vi "DARPA_DoubleJ_20220715_Arduino_ver.vi"() -> ()   [LabVIEW 2021]
uses:
  <vilib>/rvi/interface/nirviReadWriteControl/nirviReadWriteControl.xnode
  <vilib>/rvi/interface/nirviOpenFPGA/nirviOpenFPGA.xnode
  <vilib>/rvi/interface/nirviCloseFPGA/nirviCloseFPGA.xnode
  <vilib>/Instr/_visa.llb/VISA Configure Serial Port (Instr).vi
  NiFpgaLv.dll
  <vilib>/Utility/error.llb/Error Cluster From Error Code.vi
  <vilib>/rvi/interface/Simulation/niFpgaSimulationCallBeginRW.vi
  <vilib>/rvi/errors/niLvFpgaAdjustHostInterfaceError.vi
  <vilib>/FPGAPlugInAG/Dynamic/niLvFpga_Close_Dynamic.vi
  FPGA Bitfiles/darpatransitionj_FPGATarget_DARPAFPGADoubleJ_E+A750Kw4Ow.lvbitx
  DARPA_FPGA_DoubleJ_20220715.vi
  <vilib>/FPGAPlugInAG/PCIe-7857/niLvFpga_Open_PCIe-7857.vi
  <vilib>/rvi/interface/common/dynamic/niFpgaDynamicAddResources.vi
panel:
  in  "ratiocontrol":dbl
  in  "Arduino COM port":refnum<visa-resource-name>="COM7"
  in  "Shut down program 2":bool=TRUE
  in  "Initializer":bool
  out "read":string
  in  "PMT2 senstivity":bool
  in  "PMT1 senstivity":bool
  in  "Func amp":bool
  in  "Func Freq":bool
  in  "Func On time":bool
  in  "Func Delay":bool
  in  "PMT1 senstivity input":dbl caption="0.5-0.75 V"
  in  "PMT2 senstivity input":dbl caption="0.5-0.75 V"
  in  "Func amp input":dbl caption="0 - 5 V"
  in  "Func freq input":dbl caption="100 - 10k Hz"
  in  "Func on Time input":dbl caption="0.01 - 1 s"
  in  "Func delay input":dbl caption="0.01 - 1 s"
  out "PMT2 sum":u64(graph)
  out "PMT1 sum":u64(graph)
  out "Unfiltered Signal 1":i16(graph)
  out "Filtered Signal 2":i16(graph)
  out "Unfiltered Signal 2":i16(graph)
  in  "Threshold1":dbl=2.0
  in  "Threshold2":dbl=1.0
  out "LabView Timer (sec)":dbl
  out "sample diff":u64
  out "t1 (sample)":u64
  out "t0 (sample)":u64
  out "PMT1 sum":u64
  out "PMT2 sum":u64
  out "Droplet lock on":bool
  out "Filtered Signal1":dbl
  out "Filtered Signal2":dbl
  out "Droplet counter":u64
  out "Unfiltered Signal1":dbl
  out "Unfiltered Signal2":dbl
  in  "Droplet width [ms]":dbl=5.0
  in  "determine ratio (xx.xx)":dbl=1.0
  out "FPGA loop counter":u64
  out "Sorted droplet counter":u64
  out "Sort":bool
  in  "FPGA initializer":bool=TRUE
  out "FPGA timer (sec)":dbl
  out "FPGA freq":dbl
  out "LabView freq":dbl
  out "Filtered Signal 1":i16(graph)
  out "PMT1/PMT2":dbl
  out "PMT1/PMT2 (graph)":dbl(graph)
  in  "Shut down program":bool=TRUE
  in  "Set rate1":dbl=1000.0 format="%#_4g"
  in  "Units1":string(combo)="uh"
  in  "Target Vol1":dbl=1000.0 caption="Target Vol (ul)"
  in  "Direction1":string(combo)="inf"
  in  "Send1":bool
  out "Max rate1":dbl format="%#_4g"
  out "Min rate1":dbl caption="Min rate" format="%#_4g"
  in  "Pump1\nStart/Stop":bool
  out "Dispensed1":string
  in  "Reset1":bool
  out "Remains1":string
  in  "Syringe Selection1":string(combo)="BDP1MM"
  in  "dia1 (mm)":dbl=0.1 caption="Set Diameter (mm)" min=0.1 max=50.0
  out "Diameter1 (mm)":dbl
  in  "Set rate2":dbl format="%#_4g"
  in  "Units2":string(combo)="mm"
  in  "Target Vol2":dbl caption="Target Vol (ul)"
  in  "Direction2":string(combo)="inf"
  out "Max rate2":dbl format="%#_4g"
  out "Min rate2":dbl caption="Min rate" format="%#_4g"
  in  "Syringe Selection2":string(combo)="CUS"
  in  "dia2 (mm)":dbl=0.1 caption="Set Diameter (mm)" min=0.1 max=50.0
  out "Diameter2 (mm)":dbl
  in  "Set rate3":dbl format="%#_4g"
  in  "Units3":string(combo)="mm"
  in  "Target Vol3":dbl caption="Target Vol (ul)"
  in  "Direction3":string(combo)="inf"
  out "Max rate3":dbl format="%#_4g"
  out "Min rate3":dbl caption="Min rate" format="%#_4g"
  in  "Syringe Selection3":string(combo)="CUS"
  in  "dia3 (mm)":dbl=0.1 caption="Set Diameter (mm)" min=0.1 max=50.0
  out "Diameter3 (mm)":dbl
  in  "Set rate4":dbl format="%#_4g"
  in  "Units4":string(combo)="mm"
  in  "Target Vol4":dbl caption="Target Vol (ul)"
  in  "Direction4":string(combo)="inf"
  out "Max rate4":dbl format="%#_4g"
  out "Min rate4":dbl caption="Min rate" format="%#_4g"
  in  "Syringe Selection4":string(combo)="CUS"
  in  "dia4 (mm)":dbl=0.1 caption="Set Diameter (mm)" min=0.1 max=50.0
  out "Diameter4 (mm)":dbl
  in  "Pump2\nStart/Stop":bool
  in  "Pump3\nStart/Stop":bool
  in  "Pump4\nStart/Stop":bool
  out "Dispensed2":string
  out "Dispensed3":string
  out "Dispensed4":string
  out "Remains2":string
  out "Remains3":string
  out "Remains4":string
  in  "Reset2":bool
  in  "Reset3":bool
  in  "Reset4":bool
  in  "Syringe COM port":refnum<visa-resource-name>="COM3"
  out "Baud Rate":string
  in  "Output file path":string="D:\\PhD\\00TAMU\\1.research\\nanoBioSystem\\1.projects\\1.DARPA_iSENTRY\\2.src\\LabView\\transition\\FPGA7857\\output file"
  in  "file name":string="FullyAlive1"
  out "Confirm path":string
  out "Data File Ptr":refnum<file>
  # "For inner peace of developers"
  # "Communication Setting"
  # "Sorting Status"
  # "Hammamatsu display"
  # "[Pump1] Syringe Setting"
  # "[Pump2] Syringe Setting"
  # "PMT display"
  # "[Pump3] Syringe Setting"
  # "[Pump4] Syringe Setting"
  # "File saving option"
  # "Cockpit"
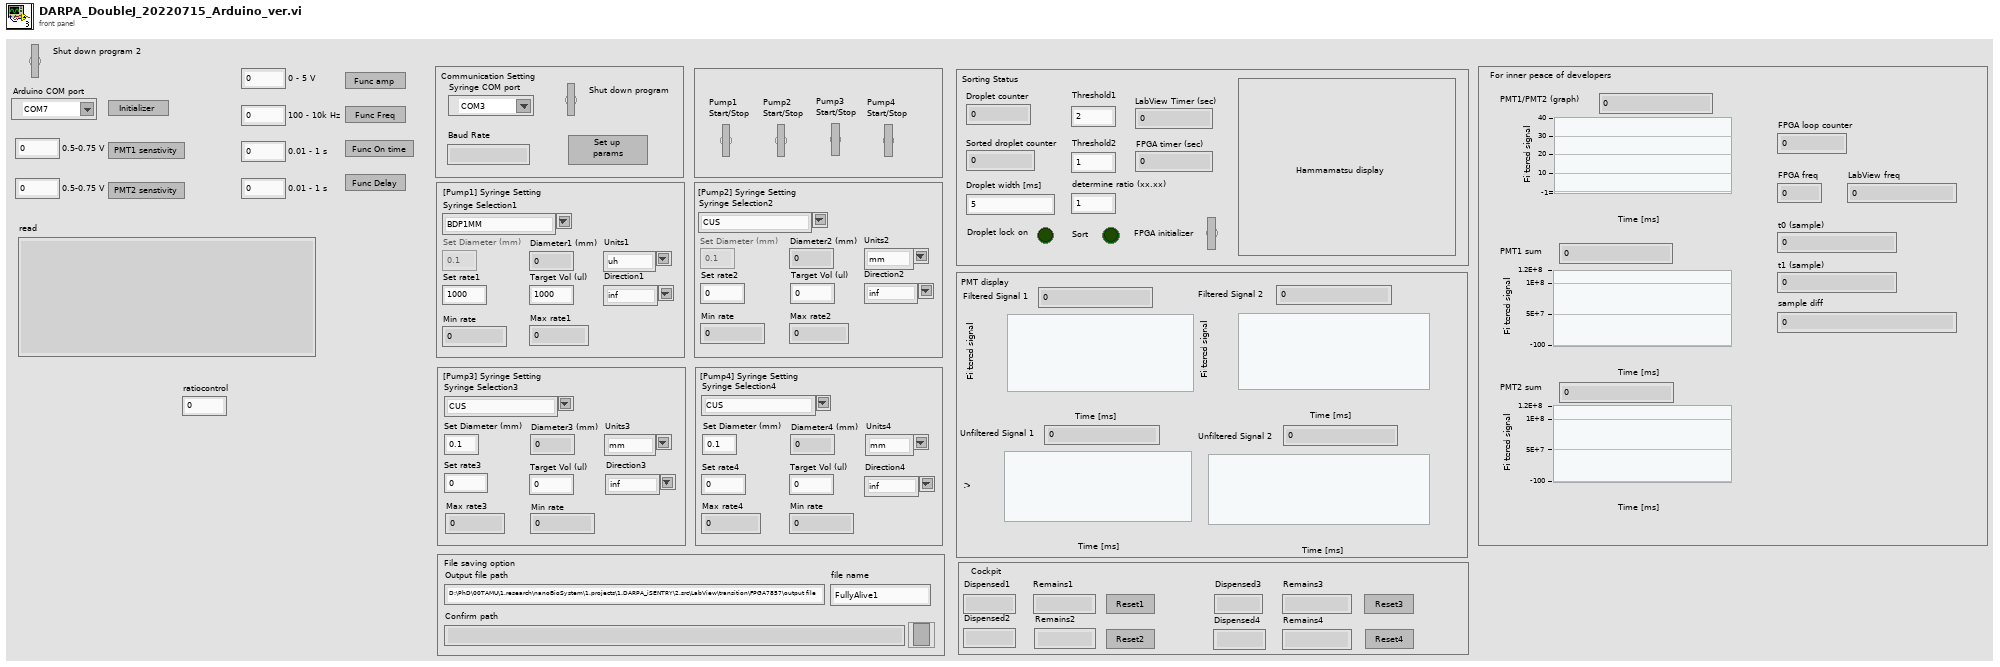
[diagram p1: front panel]
types:
  T1 = enum16{"open", "replace", "create", "open or create", "replace or create", "replace or create with confirmation"}
  T2 = enum8{"Enabled", "Disabled", "Disabled and Grayed Out"}
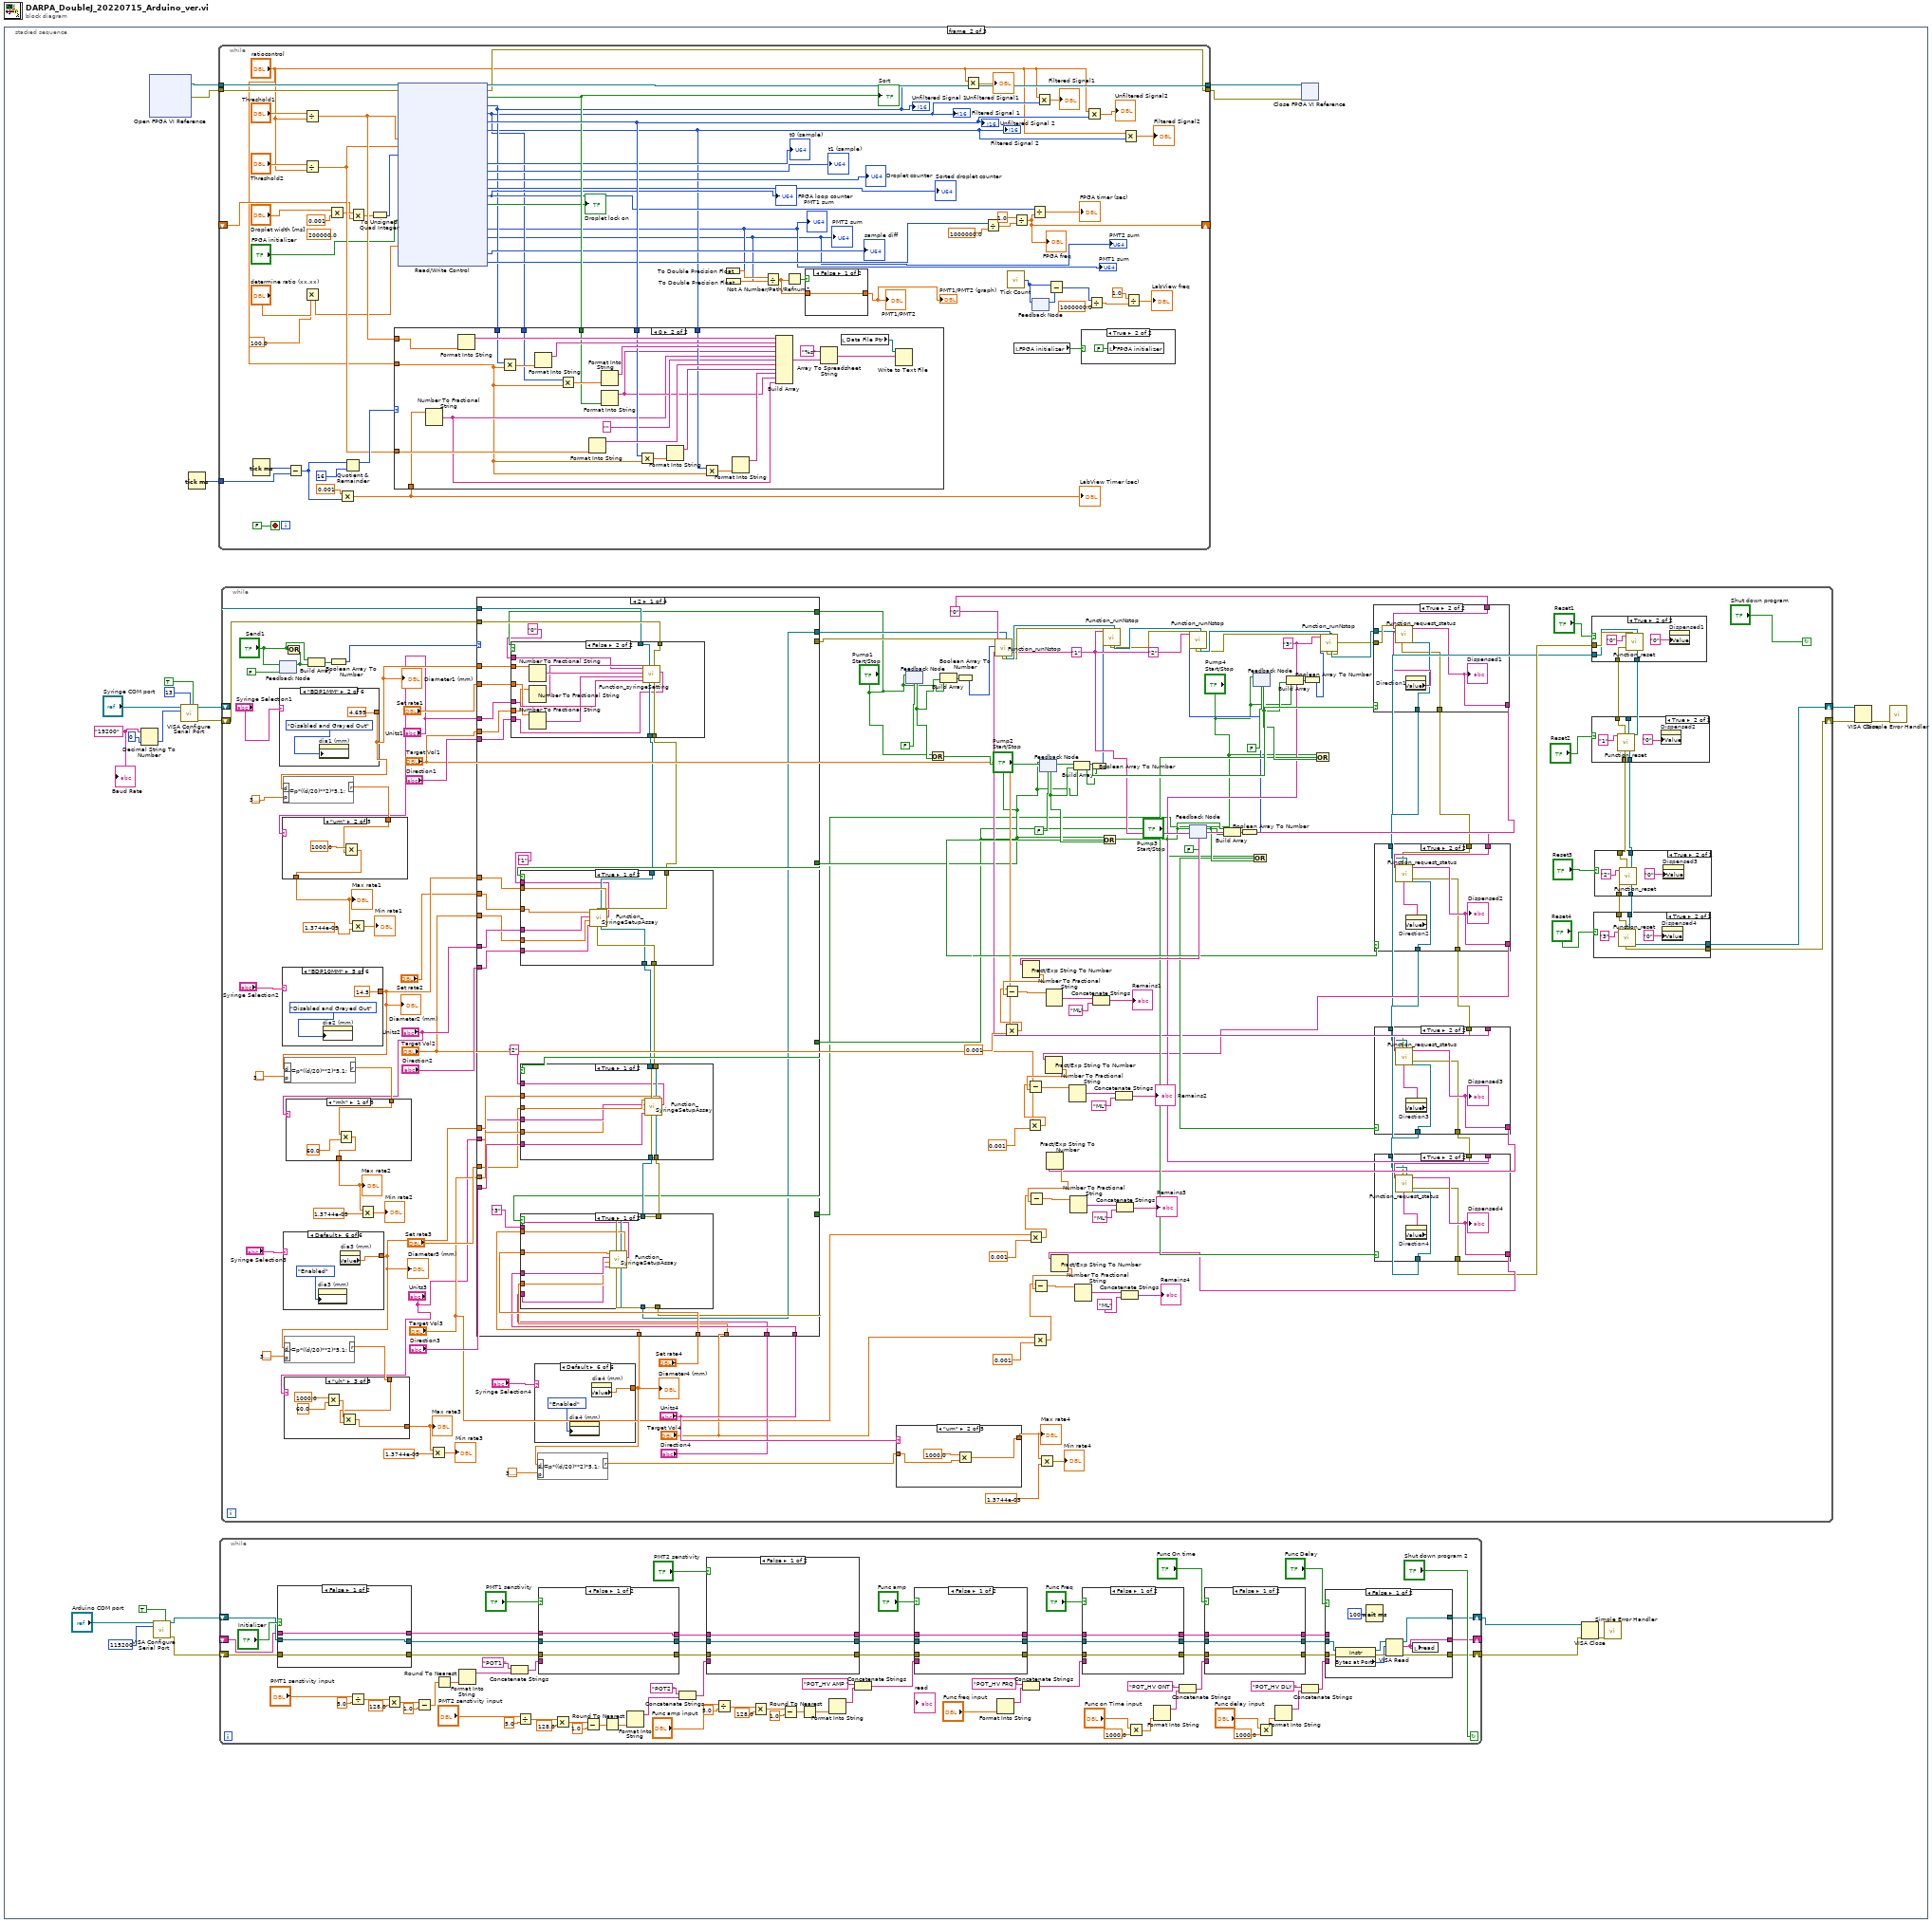
[diagram p0: block diagram]
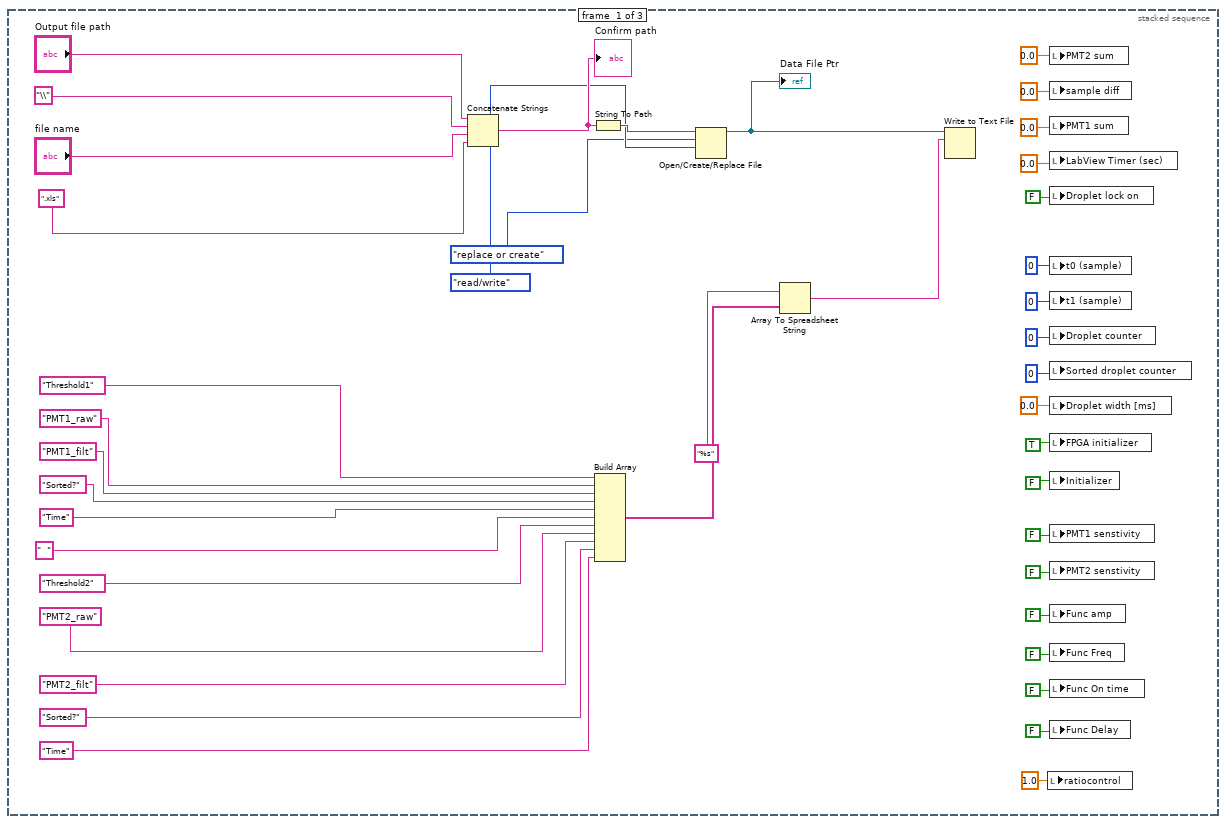
[diagram p2: hidden frame]
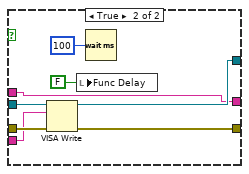
[diagram p3: hidden frame]
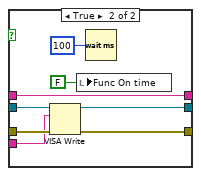
[diagram p4: hidden frame]
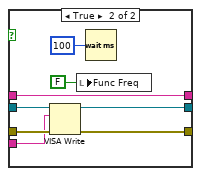
[diagram p5: hidden frame]
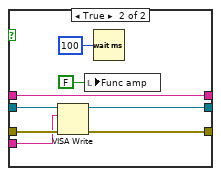
[diagram p6: hidden frame]
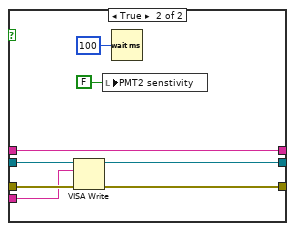
[diagram p7: hidden frame]
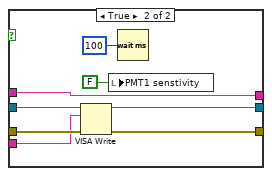
[diagram p8: hidden frame]
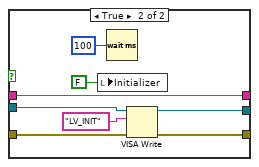
[diagram p9: hidden frame]
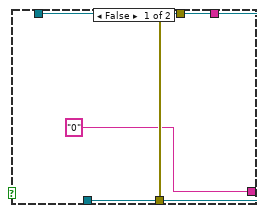
[diagram p14: hidden frame]
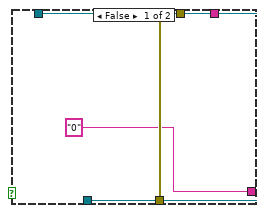
[diagram p15: hidden frame]
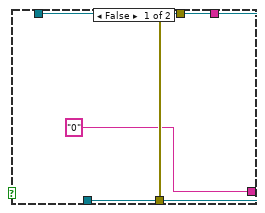
[diagram p16: hidden frame]
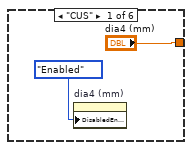
[diagram p17: hidden frame]
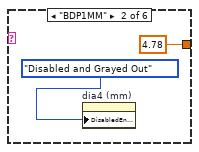
[diagram p18: hidden frame]
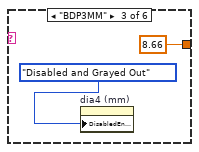
[diagram p19: hidden frame]
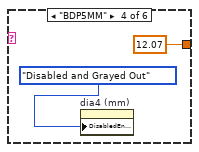
[diagram p20: hidden frame]
diagram:
  n1 = stacked-sequence {
    frame #0 {
      n2 = Concatenate Strings("Output file path", "\\" ("string"), "file name", ".xls" ("string")) -> (w41:string)
      "Confirm path" <- w41
      n3 = String To Path(string=w41) -> (path=w42:path)
      n4 = Build Array("Threshold1", "PMT1_raw", "PMT1_filt", "Sorted?", "Time", "  ", "Threshold2", "PMT2_raw", "PMT2_filt", "Sorted?", "Time") -> (w34:string[])
      n5 = Open/Create/Replace File(file path (use dialog)=w42, operation (0:open)=T1."replace or create", access (0:read/write)=enum16{"read/write", "read-only", "write-only"}."read/write") -> (refnum out=w20:refnum<file>)  [unwired: 3 in, 2 out]
      "Data File Ptr" <- w20
      n6 = Array To Spreadsheet String(array=w34, 3:"%s") -> (spreadsheet string=w22:string)  [unwired: 1 in]
      n7 = Write to Text File(file (use dialog)=w20, text=w22) -> ()  [unwired: 2 in, 3 out]
      n8 = local write "ratiocontrol"(1.0 ("ratiocontrol")) -> ()
      n9 = local write "PMT2 sum"(0.0 ("now")) -> ()
      n10 = local write "sample diff"(0.0 ("sample diff")) -> ()
      n11 = local write "PMT1 sum"(0.0 ("PMT1 sum")) -> ()
      n12 = local write "LabView Timer (sec)"(0.0 ("PMT2 sum")) -> ()
      n13 = local write "Droplet lock on"(FALSE ("Droplet lock on")) -> ()
      n14 = local write "t0 (sample)"(u64 0 ("t0 (sample)")) -> ()
      n15 = local write "t1 (sample)"(u64 0 ("t1 (sample)")) -> ()
      n16 = local write "Droplet counter"(u64 0 ("Droplet counter")) -> ()
      n17 = local write "Sorted droplet counter"(u64 0 ("Sorted droplet counter")) -> ()
      n18 = local write "Droplet width [ms]"(0.0 ("Time compensation [ms]")) -> ()
      n19 = local write "FPGA initializer"(TRUE ("FPGA initializer")) -> ()
      n20 = local write "Initializer"(FALSE ("FPGA initializer")) -> ()
      n21 = local write "PMT1 senstivity"(FALSE ("FPGA initializer")) -> ()
      n22 = local write "PMT2 senstivity"(FALSE ("FPGA initializer")) -> ()
      n23 = local write "Func amp"(FALSE ("FPGA initializer")) -> ()
      n24 = local write "Func Freq"(FALSE ("FPGA initializer")) -> ()
      n25 = local write "Func On time"(FALSE ("FPGA initializer")) -> ()
      n26 = local write "Func Delay"(FALSE ("FPGA initializer")) -> ()
    }
    frame #1 {
      w56 = "19200" ("Baud Rate")
      n27 = Decimal String To Number(string=w56, default (0L)=u32 0 ("default (0 I32)")) -> (number=w59:u32)  [unwired: 1 in, 1 out]
      n28 = xnode "Open FPGA VI Reference"() -> ("FPGA VI Reference Out"=w66:refnum<k20>, "error out"=w65:errorcluster)  [unwired: 2 in]
      n29 = call-poly "VISA Configure Serial Port"("VISA resource name"="Arduino COM port", "Enable Termination\nChar (T)"=TRUE ("Enable Termination\nChar (T)"), "baud rate (9600)"=u32 115200) -> ("VISA resource name out"=w46:refnum<visa-resource-name>, "error out"=w45:errorcluster)  [unwired: 11 in]
      n30 = call-poly "VISA Configure Serial Port"("VISA resource name"="Syringe COM port", "termination char\n(0xA = '\\n' = LF)"=u8 13 ("termination char\n(0xA = '\\n' = LF)"), "Enable Termination\nChar (T)"=TRUE ("Enable Termination\nChar (T)"), "baud rate (9600)"=w59) -> ("VISA resource name out"=w55:refnum<visa-resource-name>, "error out"=w54:errorcluster)  [unwired: 10 in]
      n31 = Tick Count (ms)() -> (millisecond timer value=w62:u32)
      n32 = while {
        tunnel: w66 -> [w744]
        tunnel: [w743] -> w64
        tunnel: w65 -> [w742]
        tunnel: [w741] -> w63
        tunnel: w62 -> [w739]
        shift-right: [w683] -> _
        shift-left: _ -> [w682]
        stop <- FALSE stop-if-true
        (unwired) 200000.0 ("y")
        n33 = Tick Count (ms)() -> (millisecond timer value=w738:u32)
        n34 = Subtract(x=w738, y=w739) -> (x-y=w733:u32)
        n35 = Divide(x="Threshold1", y="ratiocontrol") -> (x/y=w726:dbl)
        n36 = Divide(x="Threshold2", y="ratiocontrol") -> (x/y=w725:dbl)
        n37 = Multiply(x="determine ratio (xx.xx)", y=100.0) -> (x*y=w706:dbl)
        n38 = Multiply(x="Droplet width [ms]", y=0.001) -> (x*y=w708:dbl)
        n39 = Multiply(x=0.001, y=w733) -> (x*y=w700:dbl)
        "LabView Timer (sec)" <- w700
        n40 = Quotient & Remainder(x=w733, y=u32 16) -> (x-y*floor(x/y)=w735:u32)  [unwired: 1 out]
        n41 = Multiply(x=w708, y=w682) -> (x*y=w707:dbl)
        n42 = To Unsigned Quad Integer(1:w707) -> (0:w721:u64)
        n43 = xnode "Read/Write Control"("FPGA VI Reference In"=w744, "error in"=w742, "Threshold1"=w726, "Threshold2"=w725, "Time compensation [clock]"=w721, "FPGA initializer"="FPGA initializer", "determine ratio"=w706) -> ("FPGA VI Reference Out"=w743:refnum<k20>, "error out"=w741:errorcluster, "Sort"=w724:bool, "Unfiltered  Signal1"=w703:i16, "Filtered Signal1"=w691:i16, "Unfiltered  Signal2"=w727:i16, "Filtered Signal2"=w702:i16, "t0 (sample)"=→"t0 (sample)":u64, "t1 (sample)"=→"t1 (sample)":u64, "Droplet counter"=→"Droplet counter":u64, "Sorted droplet counter"=→"Sorted droplet counter":u64, "loop counter"=w712:u64, "Droplet lock on"=→"Droplet lock on":bool, "PMT1 sum"=w685:u64, "PMT2 sum"=w684:u64, "sample diff"=→"sample diff":u64, "Loop length (uSec)"=w711:u32)  [unwired: 1 out]
        "Unfiltered Signal 1" <- w703
        "Filtered Signal 2" <- w702
        "Unfiltered Signal 2" <- w727
        "PMT1 sum" <- w685
        "PMT2 sum" <- w684
        "FPGA loop counter" <- w712
        "Sort" <- w724
        "Filtered Signal 1" <- w691
        "PMT1 sum" <- w685
        "PMT2 sum" <- w684
        n44 = case shown="0" w735 {
          tunnel: w727 -> [_ w760]
          tunnel: w702 -> [_ w759]
          tunnel: w691 -> [_ w758]
          tunnel: w703 -> [_ w757]
          tunnel: w725 -> [_ w755]
          tunnel: w726 -> [_ w754]
          tunnel: w724 -> [_ w752]
          tunnel: w700 -> [_ w750]
          tunnel: "ratiocontrol" -> [_ w748]
          frame Default {
          }
          frame 0 {
            n45 = Number To Fractional String(number=w750) -> (F-format string=w749:string)  [unwired: 3 in]
            n46 = Format Into String(w754) -> (resulting string=w762:string)  [unwired: 3 in, 1 out]
            n47 = Multiply(x=w757, y=w748) -> (x*y=w770:dbl)
            n48 = Format Into String(w770) -> (resulting string=w761:string)  [unwired: 3 in, 1 out]
            n49 = Multiply(x=w758, y=w748) -> (x*y=w771:dbl)
            n50 = Format Into String(w755) -> (resulting string=w764:string)  [unwired: 3 in, 1 out]
            n51 = Format Into String(w771) -> (resulting string=w763:string)  [unwired: 3 in, 1 out]
            n52 = Format Into String(w752) -> (resulting string=w751:string)  [unwired: 3 in, 1 out]
            n53 = Multiply(x=w760, y=w748) -> (x*y=w772:dbl)
            n54 = Format Into String(w772) -> (resulting string=w765:string)  [unwired: 3 in, 1 out]
            n55 = Multiply(x=w759, y=w748) -> (x*y=w773:dbl)
            n56 = Format Into String(w773) -> (resulting string=w766:string)  [unwired: 3 in, 1 out]
            n57 = Build Array(w762, w761, w763, w751, w749, "" ("element"), w764, w765, w766, w751, w749) -> (w768:string[])
            n58 = Array To Spreadsheet String(array=w768, 3:"%s" ("format string")) -> (spreadsheet string=w767:string)  [unwired: 1 in]
            n59 = local read "Data File Ptr"() -> (w769:refnum<file>)
            n60 = Write to Text File(file (use dialog)=w769, text=w767) -> ()  [unwired: 2 in, 3 out]
          }
        }
        n61 = To Double Precision Float(number=w685) -> (double precision float=w690:dbl)
        n62 = To Double Precision Float(number=w684) -> (double precision float=w689:dbl)
        n63 = Divide(x=w690, y=w689) -> (x/y=w686:dbl)
        n64 = Not A Number/Path/Refnum?(number/path/refnum=w686) -> (NaN/Path/Refnum?=w688:bool)
        n65 = case shown="False" w688 {
          tunnel: [w745 0.0] -> w687
          tunnel: w686 -> [w745 _]
          frame False {
          }
          frame True {
          }
        }
        "PMT1/PMT2" <- w687
        "PMT1/PMT2 (graph)" <- w687
        n66 = Multiply(x="ratiocontrol", y=w703) -> (x*y=→"Unfiltered Signal1":dbl)
        n67 = Divide(x=w711, y=1000000.0 ("x")) -> (x/y=w709:dbl)
        n68 = call "Tick Count"() -> ("Tick Count(uSec)"=w693:u32)
        n69 = Divide(x=1.0, y=w709) -> (x/y=w683:dbl)
        "FPGA freq" <- w683
        n70 = local read "FPGA initializer"() -> (w713:bool)
        n71 = Divide(x=w712, y=w683) -> (x/y=→"FPGA timer (sec)":dbl)
        n72 = feedback #1() -> (w692:u32)  [unwired: 1 in]
        n73 = feedback-in #1(w693) -> ()
        n74 = Multiply(x="ratiocontrol", y=w691) -> (x*y=→"Filtered Signal1":dbl)
        n75 = Subtract(x=w693, y=w692) -> (x-y=w694:u32)
        n76 = case shown="True" w713 {
          frame False {
          }
          frame True {
            n77 = local write "FPGA initializer"(FALSE ("FPGA initializer")) -> ()
          }
        }
        n78 = Multiply(x="ratiocontrol", y=w727) -> (x*y=→"Unfiltered Signal2":dbl)
        n79 = Divide(x=w694, y=1000000.0 ("x")) -> (x/y=w697:dbl)
        n80 = Multiply(x="ratiocontrol", y=w702) -> (x*y=→"Filtered Signal2":dbl)
        n81 = Divide(x=1.0, y=w697) -> (x/y=→"LabView freq":dbl)
      }
      n82 = while {
        shift-right: [w126] -> w43
        shift-left: w46 -> [w146]
        shift-right: [w125] -> w47
        shift-left: w45 -> [w145]
        shift-right: [w127] -> _
        shift-left: _ -> [w143]
        stop <- "Shut down program 2" continue-if-true
        n83 = case shown="False" "Initializer" {
          tunnel: w146 -> [w220 w230]
          tunnel: w145 -> [w221 w229]
          tunnel: [w220 w226] -> w142
          tunnel: [w221 w225] -> w141
          tunnel: w143 -> [w222 w224]
          tunnel: [w222 w224] -> w140
          frame False {
          }
          frame True {
            n84 = local write "Initializer"(FALSE ("send")) -> ()
            n85 = Wait (ms)(milliseconds to wait=u32 100) -> ()  [unwired: 1 out]
            n86 = VISA Write(VISA resource name=w230, write buffer="LV_INIT", error in (no error)=w229) -> (VISA resource name out=w226:refnum<visa-resource-name>, error out=w225:errorcluster)  [unwired: 1 out]
          }
        }
        n87 = Divide(x="PMT1 senstivity input", y=5.0) -> (x/y=w109:dbl)
        n88 = Multiply(x=w109, y=128.0) -> (x*y=w111:dbl)
        n89 = Subtract(x=w111, y=1.0) -> (x-y=w106:dbl)
        n90 = Round To Nearest(number=w106) -> (nearest integer value=w115:dbl)
        n91 = Format Into String(w115) -> (resulting string=w114:string)  [unwired: 3 in, 1 out]
        n92 = Concatenate Strings("POT1 " ("string"), w114) -> (w112:string)
        n93 = Divide(x="PMT2 senstivity input", y=5.0) -> (x/y=w101:dbl)
        n94 = case shown="False" "PMT1 senstivity" {
          tunnel: w142 -> [w210 w219]
          tunnel: w141 -> [w209 w218]
          tunnel: [w210 w215] -> w139
          tunnel: [w209 w214] -> w138
          tunnel: w140 -> [w211 w213]
          tunnel: [w211 w213] -> w137
          tunnel: w112 -> [_ w212]
          frame False {
          }
          frame True {
            n95 = VISA Write(VISA resource name=w219, write buffer=w212, error in (no error)=w218) -> (VISA resource name out=w215:refnum<visa-resource-name>, error out=w214:errorcluster)  [unwired: 1 out]
            n96 = local write "PMT1 senstivity"(FALSE ("send")) -> ()
            n97 = Wait (ms)(milliseconds to wait=u32 100) -> ()  [unwired: 1 out]
          }
        }
        n98 = Multiply(x=w101, y=128.0) -> (x*y=w99:dbl)
        n99 = Subtract(x=w99, y=1.0) -> (x-y=w103:dbl)
        n100 = Round To Nearest(number=w103) -> (nearest integer value=w96:dbl)
        n101 = Format Into String(w96) -> (resulting string=w97:string)  [unwired: 3 in, 1 out]
        n102 = Concatenate Strings("POT2 " ("string"), w97) -> (w94:string)
        n103 = case shown="False" "PMT2 senstivity" {
          tunnel: w139 -> [w198 w208]
          tunnel: w138 -> [w199 w207]
          tunnel: [w198 w204] -> w123
          tunnel: [w199 w203] -> w122
          tunnel: w137 -> [w200 w202]
          tunnel: [w200 w202] -> w124
          tunnel: w94 -> [_ w201]
          frame False {
          }
          frame True {
            n104 = VISA Write(VISA resource name=w208, write buffer=w201, error in (no error)=w207) -> (VISA resource name out=w204:refnum<visa-resource-name>, error out=w203:errorcluster)  [unwired: 1 out]
            n105 = local write "PMT2 senstivity"(FALSE ("send")) -> ()
            n106 = Wait (ms)(milliseconds to wait=u32 100) -> ()  [unwired: 1 out]
          }
        }
        n107 = Divide(x="Func amp input", y=5.0) -> (x/y=w88:dbl)
        n108 = Multiply(x=w88, y=128.0) -> (x*y=w90:dbl)
        n109 = Subtract(x=w90, y=1.0) -> (x-y=w86:dbl)
        n110 = Round To Nearest(number=w86) -> (nearest integer value=w92:dbl)
        n111 = Format Into String(w92) -> (resulting string=w91:string)  [unwired: 3 in, 1 out]
        n112 = Concatenate Strings("POT_HV AMP " ("string"), w91) -> (w84:string)
        n113 = case shown="False" "Func amp" {
          tunnel: w123 -> [w189 w197]
          tunnel: w122 -> [w187 w196]
          tunnel: [w189 w193] -> w136
          tunnel: [w187 w192] -> w135
          tunnel: w124 -> [w188 w191]
          tunnel: [w188 w191] -> w134
          tunnel: w84 -> [_ w190]
          frame False {
          }
          frame True {
            n114 = VISA Write(VISA resource name=w197, write buffer=w190, error in (no error)=w196) -> (VISA resource name out=w193:refnum<visa-resource-name>, error out=w192:errorcluster)  [unwired: 1 out]
            n115 = local write "Func amp"(FALSE ("send")) -> ()
            n116 = Wait (ms)(milliseconds to wait=u32 100) -> ()  [unwired: 1 out]
          }
        }
        n117 = Format Into String("Func freq input") -> (resulting string=w83:string)  [unwired: 3 in, 1 out]
        n118 = Concatenate Strings("POT_HV FRQ " ("string"), w83) -> (w80:string)
        n119 = case shown="False" "Func Freq" {
          tunnel: w136 -> [w177 w186]
          tunnel: w135 -> [w176 w185]
          tunnel: [w177 w182] -> w128
          tunnel: [w176 w181] -> w129
          tunnel: w134 -> [w178 w180]
          tunnel: [w178 w180] -> w133
          tunnel: w80 -> [_ w179]
          frame False {
          }
          frame True {
            n120 = VISA Write(VISA resource name=w186, write buffer=w179, error in (no error)=w185) -> (VISA resource name out=w182:refnum<visa-resource-name>, error out=w181:errorcluster)  [unwired: 1 out]
            n121 = local write "Func Freq"(FALSE ("send")) -> ()
            n122 = Wait (ms)(milliseconds to wait=u32 100) -> ()  [unwired: 1 out]
          }
        }
        n123 = Multiply(x="Func on Time input", y=1000.0) -> (x*y=w70:dbl)
        n124 = Format Into String(w70) -> (resulting string=w79:string)  [unwired: 3 in, 1 out]
        n125 = Concatenate Strings("POT_HV ONT " ("string"), w79) -> (w78:string)
        n126 = case shown="False" "Func On time" {
          tunnel: w129 -> [w165 w175]
          tunnel: [w166 w172] -> w131
          tunnel: [w165 w171] -> w130
          tunnel: w133 -> [w167 w170]
          tunnel: [w167 w170] -> w132
          tunnel: w128 -> [w166 w169]
          tunnel: w78 -> [_ w168]
          frame False {
          }
          frame True {
            n127 = VISA Write(VISA resource name=w169, write buffer=w168, error in (no error)=w175) -> (VISA resource name out=w172:refnum<visa-resource-name>, error out=w171:errorcluster)  [unwired: 1 out]
            n128 = local write "Func On time"(FALSE ("send")) -> ()
            n129 = Wait (ms)(milliseconds to wait=u32 100) -> ()  [unwired: 1 out]
          }
        }
        n130 = Multiply(x="Func delay input", y=1000.0) -> (x*y=w68:dbl)
        n131 = Format Into String(w68) -> (resulting string=w77:string)  [unwired: 3 in, 1 out]
        n132 = Concatenate Strings("POT_HV DLY " ("string"), w77) -> (w76:string)
        n133 = case shown="False" "Func Delay" {
          tunnel: w131 -> [w153 w164]
          tunnel: w130 -> [w152 w163]
          tunnel: [w151 w160] -> w126
          tunnel: [w150 w159] -> w125
          tunnel: w132 -> [_ w158]
          tunnel: [w149 w158] -> w127
          tunnel: w76 -> [_ w157]
          frame False {
            n134 = property class="Instr"(reference=w153, error in=w152) -> (reference out=w154:refnum<visa-resource-name>, error out=w156:errorcluster, "Bytes at Port"=w155:u32)
            n135 = Wait (ms)(milliseconds to wait=u32 100) -> ()  [unwired: 1 out]
            n136 = VISA Read(VISA resource name=w154, byte count=w155, error in (no error)=w156) -> (VISA resource name out=w151:refnum<visa-resource-name>, read buffer=w149:string, error out=w150:errorcluster)  [unwired: 1 out]
            n137 = local write "read"(w149) -> ()
          }
          frame True {
            n138 = VISA Write(VISA resource name=w164, write buffer=w157, error in (no error)=w163) -> (VISA resource name out=w160:refnum<visa-resource-name>, error out=w159:errorcluster)  [unwired: 1 out]
            n139 = local write "Func Delay"(FALSE ("send")) -> ()
            n140 = Wait (ms)(milliseconds to wait=u32 100) -> ()  [unwired: 1 out]
          }
        }
      }
      n141 = while {
        shift-right: [w232] -> w52
        shift-left: w55 -> [w234]
        shift-right: [w231] -> w51
        shift-left: w54 -> [w233]
        stop <- "Shut down program" continue-if-true
        w285 = "3" ("trimmed string")
        w286 = "2" ("trimmed string")
        w294 = "1" ("trimmed string")
        w314 = "0" ("trimmed string")
        n142 = case shown="\"BDP1MM\"" "Syringe Selection1" {
          tunnel: ["dia1 (mm)" 4.699 ("dia (mm)") 8.66 ("dia (mm)") 12.07 ("dia (mm)") 14.5 ("dia (mm)") w521] -> w345
          frame "CUS" {
            n143 = property on="dia1 (mm)" class="DigNum (strict)"("DisabledEnum"=T2."Enabled" ("Disabled")) -> ()  [unwired: 2 in, 2 out]
          }
          frame "BDP1MM" {
            n144 = property on="dia1 (mm)" class="DigNum (strict)"("DisabledEnum"=T2."Disabled and Grayed Out" ("Disabled")) -> ()  [unwired: 2 in, 2 out]
          }
          frame "BDP3MM" {
            n145 = property on="dia1 (mm)" class="DigNum (strict)"("DisabledEnum"=T2."Disabled and Grayed Out" ("Disabled")) -> ()  [unwired: 2 in, 2 out]
          }
          frame "BDP5MM" {
            n146 = property on="dia1 (mm)" class="DigNum (strict)"("DisabledEnum"=T2."Disabled and Grayed Out" ("Disabled")) -> ()  [unwired: 2 in, 2 out]
          }
          frame "BDP10MM" {
            n147 = property on="dia1 (mm)" class="DigNum (strict)"("DisabledEnum"=T2."Disabled and Grayed Out" ("Disabled")) -> ()  [unwired: 2 in, 2 out]
          }
          frame Default {
            n148 = property on="dia1 (mm)" class="DigNum (strict)"("DisabledEnum"=T2."Enabled" ("Disabled")) -> ()  [unwired: 2 in, 2 out]
            n149 = property on="dia1 (mm)" class="DigNum (strict)"() -> ("Value"=w521:dbl)  [unwired: 2 in, 2 out]
          }
        }
        "Diameter1 (mm)" <- w345
        n150 = feedback #2(FALSE ("Go 1")) -> (w359:bool)
        n151 = feedback-in #2("Send1") -> ()
        n152 = case shown="\"BDP10MM\"" "Syringe Selection2" {
          tunnel: ["dia2 (mm)" 4.78 ("dia (mm)") 8.66 ("dia (mm)") 12.07 ("dia (mm)") 14.5 ("dia (mm)") w496] -> w337
          frame "CUS" {
            n153 = property on="dia2 (mm)" class="DigNum (strict)"("DisabledEnum"=T2."Enabled" ("Disabled")) -> ()  [unwired: 2 in, 2 out]
          }
          frame "BDP1MM" {
            n154 = property on="dia2 (mm)" class="DigNum (strict)"("DisabledEnum"=T2."Disabled and Grayed Out" ("Disabled")) -> ()  [unwired: 2 in, 2 out]
          }
          frame "BDP3MM" {
            n155 = property on="dia2 (mm)" class="DigNum (strict)"("DisabledEnum"=T2."Disabled and Grayed Out" ("Disabled")) -> ()  [unwired: 2 in, 2 out]
          }
          frame "BDP5MM" {
            n156 = property on="dia2 (mm)" class="DigNum (strict)"("DisabledEnum"=T2."Disabled and Grayed Out" ("Disabled")) -> ()  [unwired: 2 in, 2 out]
          }
          frame "BDP10MM" {
            n157 = property on="dia2 (mm)" class="DigNum (strict)"("DisabledEnum"=T2."Disabled and Grayed Out" ("Disabled")) -> ()  [unwired: 2 in, 2 out]
          }
          frame Default {
            n158 = property on="dia2 (mm)" class="DigNum (strict)"("DisabledEnum"=T2."Enabled" ("Disabled")) -> ()  [unwired: 2 in, 2 out]
            n159 = property on="dia2 (mm)" class="DigNum (strict)"() -> ("Value"=w496:dbl)  [unwired: 2 in, 2 out]
          }
        }
        "Diameter2 (mm)" <- w337
        n160 = formula code="r=p*((d/20)**2)*5.1;"("d"=w345, "p"=3.141592653589793) -> ("r"=w364:dbl)
        n161 = case shown="\"um\"" "Units1" {
          tunnel: w364 -> [w533 w535 w539 w543 w544]
          tunnel: [w532 w536 w538 w543 w544] -> w365
          frame "mh" {
            n162 = Multiply(x=w533, y=60.0) -> (x*y=w532:dbl)
          }
          frame "um" {
            n163 = Multiply(x=1000.0, y=w535) -> (x*y=w536:dbl)
          }
          frame "uh" {
            n164 = Multiply(x=1000.0, y=60.0) -> (x*y=w542:dbl)
            n165 = Multiply(x=w542, y=w539) -> (x*y=w538:dbl)
          }
          frame Default {
          }
          frame "mm" {
          }
        }
        "Max rate1" <- w365
        n166 = case shown="Default" "Syringe Selection3" {
          tunnel: ["dia3 (mm)" 4.78 ("dia (mm)") 8.66 ("dia (mm)") 12.07 ("dia (mm)") 14.5 ("dia (mm)") w471] -> w327
          frame "CUS" {
            n167 = property on="dia3 (mm)" class="DigNum (strict)"("DisabledEnum"=T2."Enabled" ("Disabled")) -> ()  [unwired: 2 in, 2 out]
          }
          frame "BDP1MM" {
            n168 = property on="dia3 (mm)" class="DigNum (strict)"("DisabledEnum"=T2."Disabled and Grayed Out" ("Disabled")) -> ()  [unwired: 2 in, 2 out]
          }
          frame "BDP3MM" {
            n169 = property on="dia3 (mm)" class="DigNum (strict)"("DisabledEnum"=T2."Disabled and Grayed Out" ("Disabled")) -> ()  [unwired: 2 in, 2 out]
          }
          frame "BDP5MM" {
            n170 = property on="dia3 (mm)" class="DigNum (strict)"("DisabledEnum"=T2."Disabled and Grayed Out" ("Disabled")) -> ()  [unwired: 2 in, 2 out]
          }
          frame "BDP10MM" {
            n171 = property on="dia3 (mm)" class="DigNum (strict)"("DisabledEnum"=T2."Disabled and Grayed Out" ("Disabled")) -> ()  [unwired: 2 in, 2 out]
          }
          frame Default {
            n172 = property on="dia3 (mm)" class="DigNum (strict)"("DisabledEnum"=T2."Enabled" ("Disabled")) -> ()  [unwired: 2 in, 2 out]
            n173 = property on="dia3 (mm)" class="DigNum (strict)"() -> ("Value"=w471:dbl)  [unwired: 2 in, 2 out]
          }
        }
        "Diameter3 (mm)" <- w327
        n174 = formula code="r=p*((d/20)**2)*5.1;"("d"=w327, "p"=3.141592653589793) -> ("r"=w329:dbl)
        n175 = case shown="\"uh\"" "Units3" {
          tunnel: w329 -> [w473 w475 w479 w483 w484]
          tunnel: [w472 w476 w478 w483 w484] -> w330
          frame "mh" {
            n176 = Multiply(x=w473, y=60.0) -> (x*y=w472:dbl)
          }
          frame "um" {
            n177 = Multiply(x=1000.0, y=w475) -> (x*y=w476:dbl)
          }
          frame "uh" {
            n178 = Multiply(x=1000.0, y=60.0) -> (x*y=w482:dbl)
            n179 = Multiply(x=w482, y=w479) -> (x*y=w478:dbl)
          }
          frame Default {
          }
          frame "mm" {
          }
        }
        "Max rate3" <- w330
        n180 = formula code="r=p*((d/20)**2)*5.1;"("d"=w337, "p"=3.141592653589793) -> ("r"=w339:dbl)
        n181 = Or(x="Send1", y=w359) -> ()  [unwired: 1 out]
        n182 = case shown="\"mh\"" "Units2" {
          tunnel: w339 -> [w498 w500 w504 w508 w509]
          tunnel: [w497 w501 w503 w508 w509] -> w340
          frame "mh" {
            n183 = Multiply(x=w498, y=60.0) -> (x*y=w497:dbl)
          }
          frame "um" {
            n184 = Multiply(x=1000.0, y=w500) -> (x*y=w501:dbl)
          }
          frame "uh" {
            n185 = Multiply(x=1000.0, y=60.0) -> (x*y=w507:dbl)
            n186 = Multiply(x=w507, y=w504) -> (x*y=w503:dbl)
          }
          frame Default {
          }
          frame "mm" {
          }
        }
        "Max rate2" <- w340
        n187 = Build Array("Send1", w359) -> (w362:bool[])
        n188 = Boolean Array To Number(Boolean array=w362) -> (number=w360:u32)
        n189 = Multiply(x=w365, y=1.3744e-05) -> (x*y=→"Min rate1":dbl)
        n190 = Multiply(x=w340, y=1.3744e-05) -> (x*y=→"Min rate2":dbl)
        n191 = Multiply(x=w330, y=1.3744e-05) -> (x*y=→"Min rate3":dbl)
        n192 = case shown="Default" "Syringe Selection4" {
          tunnel: ["dia4 (mm)" 4.78 ("dia (mm)") 8.66 ("dia (mm)") 12.07 ("dia (mm)") 14.5 ("dia (mm)") w446] -> w318
          frame "CUS" {
            n193 = property on="dia4 (mm)" class="DigNum (strict)"("DisabledEnum"=T2."Enabled" ("Disabled")) -> ()  [unwired: 2 in, 2 out]
          }
          frame "BDP1MM" {
            n194 = property on="dia4 (mm)" class="DigNum (strict)"("DisabledEnum"=T2."Disabled and Grayed Out" ("Disabled")) -> ()  [unwired: 2 in, 2 out]
          }
          frame "BDP3MM" {
            n195 = property on="dia4 (mm)" class="DigNum (strict)"("DisabledEnum"=T2."Disabled and Grayed Out" ("Disabled")) -> ()  [unwired: 2 in, 2 out]
          }
          frame "BDP5MM" {
            n196 = property on="dia4 (mm)" class="DigNum (strict)"("DisabledEnum"=T2."Disabled and Grayed Out" ("Disabled")) -> ()  [unwired: 2 in, 2 out]
          }
          frame "BDP10MM" {
            n197 = property on="dia4 (mm)" class="DigNum (strict)"("DisabledEnum"=T2."Disabled and Grayed Out" ("Disabled")) -> ()  [unwired: 2 in, 2 out]
          }
          frame Default {
            n198 = property on="dia4 (mm)" class="DigNum (strict)"("DisabledEnum"=T2."Enabled" ("Disabled")) -> ()  [unwired: 2 in, 2 out]
            n199 = property on="dia4 (mm)" class="DigNum (strict)"() -> ("Value"=w446:dbl)  [unwired: 2 in, 2 out]
          }
        }
        "Diameter4 (mm)" <- w318
        n200 = case shown="2" w360 {
          tunnel: w234 -> [w580 w675 w678 w679]
          tunnel: w233 -> [w581 w676 w677 w680]
          tunnel: [w546 w676 w677 w680] -> w313
          tunnel: [w545 w675 w678 w679] -> w312
          tunnel: w345 -> [w577 _ _ _]
          tunnel: "Set rate1" -> [w576 _ _ _]
          tunnel: "Units1" -> [w579 _ _ _]
          tunnel: "Target Vol1" -> [w578 _ _ _]
          tunnel: "Direction1" -> [w582 _ _ _]
          tunnel: w337 -> [w572 _ _ _]
          tunnel: "Set rate2" -> [w571 _ _ _]
          tunnel: "Units2" -> [w568 _ _ _]
          tunnel: "Target Vol2" -> [w567 _ _ _]
          tunnel: "Direction2" -> [w566 _ _ _]
          tunnel: w327 -> [w560 _ _ _]
          tunnel: "Set rate3" -> [w556 _ _ _]
          tunnel: "Units3" -> [w557 _ _ _]
          tunnel: "Direction3" -> [w559 _ _ _]
          tunnel: "Target Vol3" -> [w558 _ _ _]
          tunnel: w318 -> [w552 _ _ _]
          tunnel: "Set rate4" -> [w551 _ _ _]
          tunnel: "Units4" -> [w550 _ _ _]
          tunnel: "Target Vol4" -> [w549 _ _ _]
          tunnel: "Direction4" -> [w548 _ _ _]
          tunnel: "Pump1\nStart/Stop" -> [w575 _ _ _]
          tunnel: "Pump2\nStart/Stop" -> [w573 _ _ _]
          tunnel: "Pump3\nStart/Stop" -> [w563 _ _ _]
          tunnel: "Pump4\nStart/Stop" -> [w547 _ _ _]
          frame 2 {
            n201 = case shown="False" w575 {
              tunnel: w582 -> [w653 w669]
              tunnel: w581 -> [w661 w674]
              tunnel: w580 -> [w656 w673]
              tunnel: w579 -> [w655 w670]
              tunnel: w578 -> [w654 w664]
              tunnel: w577 -> [w658 w668]
              tunnel: w576 -> [w657 w666]
              tunnel: [w660 w671] -> w570
              tunnel: [w659 w672] -> w569
              tunnel: "0" ("Pump Add") -> [w652 w662]
              frame True {
                n202 = call "Function_SyringeSetupAssay.vi"("PumpID"=w652, "Diameter (mm)"=w658, "VISA resource name in"=w656, "error in"=w661, "Direction"=w653, "Target Vol1"=w654, "Units"=w655, "Set rate"=w657) -> ("VISA resource name out"=w659:refnum<visa-resource-name>, "error out"=w660:errorcluster)  [unwired: 2 in]
              }
              frame False {
                n203 = Number To Fractional String(number=w668) -> (F-format string=w667:string)  [unwired: 3 in]
                n204 = Number To Fractional String(number=w664) -> (F-format string=w663:string)  [unwired: 3 in]
                n205 = Number To Fractional String(number=w666) -> (F-format string=w665:string)  [unwired: 3 in]
                n206 = call "Function_syringeSetting.vi"("Direction"=w669, "target volume- string"=w663, "error in"=w674, "VISA resource name in"=w673, "units"=w670, "set rate- string"=w665, "diameter(mm)-string"=w667, "address (string)"=w662) -> ("error out"=w671:errorcluster, "VISA resource name out"=w672:refnum<visa-resource-name>)  [unwired: 2 in]
              }
            }
            n207 = case shown="True" w573 {
              tunnel: w566 -> [w630 w646]
              tunnel: w570 -> [w638 w651]
              tunnel: w569 -> [w633 w650]
              tunnel: w568 -> [w632 w647]
              tunnel: w567 -> [w631 w641]
              tunnel: w572 -> [w635 w645]
              tunnel: w571 -> [w634 w643]
              tunnel: [w637 w648] -> w561
              tunnel: [w636 w649] -> w562
              tunnel: "1" ("Pump Add") -> [w629 w639]
              frame True {
                n208 = call "Function_SyringeSetupAssay.vi"("PumpID"=w629, "Diameter (mm)"=w635, "VISA resource name in"=w633, "error in"=w638, "Direction"=w630, "Target Vol1"=w631, "Units"=w632, "Set rate"=w634) -> ("VISA resource name out"=w636:refnum<visa-resource-name>, "error out"=w637:errorcluster)  [unwired: 2 in]
              }
              frame False {
                n209 = Number To Fractional String(number=w641) -> (F-format string=w640:string)  [unwired: 3 in]
                n210 = Number To Fractional String(number=w645) -> (F-format string=w644:string)  [unwired: 3 in]
                n211 = Number To Fractional String(number=w643) -> (F-format string=w642:string)  [unwired: 3 in]
                n212 = call "Function_syringeSetting.vi"("Direction"=w646, "target volume- string"=w640, "error in"=w651, "VISA resource name in"=w650, "units"=w647, "set rate- string"=w642, "diameter(mm)-string"=w644, "address (string)"=w639) -> ("error out"=w648:errorcluster, "VISA resource name out"=w649:refnum<visa-resource-name>)  [unwired: 2 in]
              }
            }
            n213 = case shown="True" w563 {
              tunnel: w559 -> [w607 w624]
              tunnel: w561 -> [w615 w628]
              tunnel: w562 -> [w610 w616]
              tunnel: w557 -> [w609 w625]
              tunnel: w558 -> [w608 w619]
              tunnel: w560 -> [w612 w623]
              tunnel: w556 -> [w611 w621]
              tunnel: [w614 w626] -> w554
              tunnel: [w613 w627] -> w553
              tunnel: "2" ("Pump Add") -> [w606 w617]
              frame True {
                n214 = call "Function_SyringeSetupAssay.vi"("PumpID"=w606, "Diameter (mm)"=w612, "VISA resource name in"=w610, "error in"=w615, "Direction"=w607, "Target Vol1"=w608, "Units"=w609, "Set rate"=w611) -> ("VISA resource name out"=w613:refnum<visa-resource-name>, "error out"=w614:errorcluster)  [unwired: 2 in]
              }
              frame False {
                n215 = Number To Fractional String(number=w619) -> (F-format string=w618:string)  [unwired: 3 in]
                n216 = Number To Fractional String(number=w623) -> (F-format string=w622:string)  [unwired: 3 in]
                n217 = Number To Fractional String(number=w621) -> (F-format string=w620:string)  [unwired: 3 in]
                n218 = call "Function_syringeSetting.vi"("Direction"=w624, "target volume- string"=w618, "error in"=w628, "VISA resource name in"=w616, "units"=w625, "set rate- string"=w620, "diameter(mm)-string"=w622, "address (string)"=w617) -> ("error out"=w626:errorcluster, "VISA resource name out"=w627:refnum<visa-resource-name>)  [unwired: 2 in]
              }
            }
            n219 = case shown="True" w547 {
              tunnel: w548 -> [w584 w600]
              tunnel: w554 -> [w592 w605]
              tunnel: w553 -> [w587 w604]
              tunnel: w550 -> [w586 w601]
              tunnel: w549 -> [w585 w595]
              tunnel: w552 -> [w589 w599]
              tunnel: w551 -> [w588 w597]
              tunnel: [w591 w602] -> w546
              tunnel: [w590 w603] -> w545
              tunnel: "3" ("Pump Add") -> [w583 w593]
              frame True {
                n220 = call "Function_SyringeSetupAssay.vi"("PumpID"=w583, "Diameter (mm)"=w589, "VISA resource name in"=w587, "error in"=w592, "Direction"=w584, "Target Vol1"=w585, "Units"=w586, "Set rate"=w588) -> ("VISA resource name out"=w590:refnum<visa-resource-name>, "error out"=w591:errorcluster)  [unwired: 2 in]
              }
              frame False {
                n221 = Number To Fractional String(number=w595) -> (F-format string=w594:string)  [unwired: 3 in]
                n222 = Number To Fractional String(number=w599) -> (F-format string=w598:string)  [unwired: 3 in]
                n223 = Number To Fractional String(number=w597) -> (F-format string=w596:string)  [unwired: 3 in]
                n224 = call "Function_syringeSetting.vi"("Direction"=w600, "target volume- string"=w594, "error in"=w605, "VISA resource name in"=w604, "units"=w601, "set rate- string"=w596, "diameter(mm)-string"=w598, "address (string)"=w593) -> ("error out"=w602:errorcluster, "VISA resource name out"=w603:refnum<visa-resource-name>)  [unwired: 2 in]
              }
            }
          }
          frame 1 {
          }
          frame Default {
          }
          frame 3 {
          }
        }
        n225 = formula code="r=p*((d/20)**2)*5.1;"("d"=w318, "p"=3.141592653589793) -> ("r"=w320:dbl)
        n226 = case shown="\"um\"" "Units4" {
          tunnel: w320 -> [w448 w450 w454 w458 w459]
          tunnel: [w447 w451 w453 w458 w459] -> w321
          frame "mh" {
            n227 = Multiply(x=w448, y=60.0) -> (x*y=w447:dbl)
          }
          frame "um" {
            n228 = Multiply(x=1000.0, y=w450) -> (x*y=w451:dbl)
          }
          frame "uh" {
            n229 = Multiply(x=1000.0, y=60.0) -> (x*y=w457:dbl)
            n230 = Multiply(x=w457, y=w454) -> (x*y=w453:dbl)
          }
          frame Default {
          }
          frame "mm" {
          }
        }
        "Max rate4" <- w321
        n231 = feedback #3(FALSE ("Motor Start/Stop")) -> (w357:bool)
        n232 = feedback-in #3("Pump1\nStart/Stop") -> ()
        n233 = Or(x="Pump1\nStart/Stop", y=w357) -> (x .or. y?=w356:bool)
        n234 = Build Array("Pump1\nStart/Stop", w357) -> (w371:bool[])
        n235 = Boolean Array To Number(Boolean array=w371) -> (number=w245:u32)
        n236 = call "Function_runNstop.vi"("VISA resource name in"=w312, "error in"=w313, "condition"=w245, "Server addr"=w314) -> ("VISA resource name out"=w308:refnum<visa-resource-name>, "error out"=w307:errorcluster)  [unwired: 6 in]
        n237 = Multiply(x="Target Vol1", y=0.001) -> (x*y=w350:dbl)
        n238 = Multiply(x="Target Vol2", y=0.001) -> (x*y=w281:dbl)
        n239 = Multiply(x="Target Vol3", y=0.001) -> (x*y=w274:dbl)
        n240 = Multiply(x="Target Vol4", y=0.001) -> (x*y=w267:dbl)
        n241 = Multiply(x=w321, y=1.3744e-05) -> (x*y=→"Min rate4":dbl)
        n242 = feedback #4(FALSE ("Motor Start/Stop")) -> (w309:bool)
        n243 = feedback-in #4("Pump2\nStart/Stop") -> ()
        n244 = Build Array("Pump2\nStart/Stop", w309) -> (w311:bool[])
        n245 = Boolean Array To Number(Boolean array=w311) -> (number=w244:u32)
        n246 = Or(x="Pump2\nStart/Stop", y=w309) -> (x .or. y?=w291:bool)
        n247 = call "Function_runNstop.vi"("VISA resource name in"=w308, "error in"=w307, "condition"=w244, "Server addr"=w294) -> ("VISA resource name out"=w300:refnum<visa-resource-name>, "error out"=w237:errorcluster)  [unwired: 6 in]
        n248 = feedback #5(FALSE ("Motor Start/Stop")) -> (w304:bool)
        n249 = feedback-in #5("Pump3\nStart/Stop") -> ()
        n250 = Build Array("Pump3\nStart/Stop", w304) -> (w306:bool[])
        n251 = Boolean Array To Number(Boolean array=w306) -> (number=w243:u32)
        n252 = call "Function_runNstop.vi"("VISA resource name in"=w300, "error in"=w237, "condition"=w243, "Server addr"=w286) -> ("VISA resource name out"=w299:refnum<visa-resource-name>, "error out"=w236:errorcluster)  [unwired: 6 in]
        n253 = Or(x="Pump3\nStart/Stop", y=w304) -> (x .or. y?=w290:bool)
        n254 = feedback #6(FALSE ("Motor Start/Stop")) -> (w301:bool)
        n255 = feedback-in #6("Pump4\nStart/Stop") -> ()
        n256 = Build Array("Pump4\nStart/Stop", w301) -> (w303:bool[])
        n257 = Boolean Array To Number(Boolean array=w303) -> (number=w242:u32)
        n258 = Or(x="Pump4\nStart/Stop", y=w301) -> (x .or. y?=w289:bool)
        n259 = call "Function_runNstop.vi"("VISA resource name in"=w299, "error in"=w236, "condition"=w242, "Server addr"=w285) -> ("VISA resource name out"=w298:refnum<visa-resource-name>, "error out"=w297:errorcluster)  [unwired: 6 in]
        n260 = case shown="True" w356 {
          tunnel: [w524 w527] -> w296
          tunnel: [w523 w526] -> w295
          tunnel: w298 -> [w524 w525]
          tunnel: w297 -> [w523 w529]
          tunnel: w314 -> [_ w530]
          tunnel: ["0" ("Vol Infused") w528] -> w355
          frame False {
          }
          frame True {
            n261 = property on="Direction1" class="CmbBox"() -> ("Value"=w531:string)  [unwired: 2 in, 2 out]
            n262 = call "Function_request_status.vi"("VISA resource name in"=w525, "error in"=w529, "Direction"=w531, "Server addr"=w530) -> ("Dispensed1"=w528:string, "VISA resource name out"=w527:refnum<visa-resource-name>, "error out"=w526:errorcluster)  [unwired: 5 in]
            "Dispensed1" <- w528
          }
        }
        n263 = Fract/Exp String To Number(string=w355) -> (number=w354:dbl)  [unwired: 3 in, 1 out]
        n264 = Subtract(x=w350, y=w354) -> (x-y=w353:dbl)
        n265 = Number To Fractional String(number=w353) -> (F-format string=w349:string)  [unwired: 3 in]
        n266 = Concatenate Strings(w349, "ML" ("string")) -> (→"Remains1":string)
        n267 = case shown="True" w291 {
          tunnel: [w427 w429] -> w293
          tunnel: [w426 w428] -> w292
          tunnel: w296 -> [w427 w432]
          tunnel: w295 -> [w426 w431]
          tunnel: w294 -> [_ w433]
          tunnel: ["0" ("Vol Infused") w430] -> w260
          frame False {
          }
          frame True {
            n268 = property on="Direction2" class="CmbBox"() -> ("Value"=w434:string)  [unwired: 2 in, 2 out]
            n269 = call "Function_request_status.vi"("VISA resource name in"=w432, "error in"=w431, "Direction"=w434, "Server addr"=w433) -> ("Dispensed1"=w430:string, "VISA resource name out"=w429:refnum<visa-resource-name>, "error out"=w428:errorcluster)  [unwired: 5 in]
            "Dispensed2" <- w430
          }
        }
        n270 = Fract/Exp String To Number(string=w260) -> (number=w284:dbl)  [unwired: 3 in, 1 out]
        n271 = Subtract(x=w281, y=w284) -> (x-y=w283:dbl)
        n272 = Number To Fractional String(number=w283) -> (F-format string=w280:string)  [unwired: 3 in]
        n273 = Concatenate Strings(w280, "ML" ("string")) -> (→"Remains2":string)
        n274 = case shown="True" w290 {
          tunnel: [w417 w419] -> w288
          tunnel: [w416 w418] -> w287
          tunnel: w293 -> [w417 w422]
          tunnel: w292 -> [w416 w421]
          tunnel: w286 -> [_ w423]
          tunnel: ["0" ("Vol Infused") w420] -> w259
          frame False {
          }
          frame True {
            n275 = property on="Direction3" class="CmbBox"() -> ("Value"=w424:string)  [unwired: 2 in, 2 out]
            n276 = call "Function_request_status.vi"("VISA resource name in"=w422, "error in"=w421, "Direction"=w424, "Server addr"=w423) -> ("Dispensed1"=w420:string, "VISA resource name out"=w419:refnum<visa-resource-name>, "error out"=w418:errorcluster)  [unwired: 5 in]
            "Dispensed3" <- w420
          }
        }
        n277 = Fract/Exp String To Number(string=w259) -> (number=w277:dbl)  [unwired: 3 in, 1 out]
        n278 = Subtract(x=w274, y=w277) -> (x-y=w276:dbl)
        n279 = Number To Fractional String(number=w276) -> (F-format string=w273:string)  [unwired: 3 in]
        n280 = Concatenate Strings(w273, "ML" ("string")) -> (→"Remains3":string)
        n281 = case shown="True" w289 {
          tunnel: [w407 w409] -> w255
          tunnel: [w406 w408] -> w256
          tunnel: w288 -> [w407 w412]
          tunnel: w287 -> [w406 w411]
          tunnel: w285 -> [_ w413]
          tunnel: ["0" ("Vol Infused") w410] -> w258
          frame False {
          }
          frame True {
            n282 = property on="Direction4" class="CmbBox"() -> ("Value"=w414:string)  [unwired: 2 in, 2 out]
            n283 = call "Function_request_status.vi"("VISA resource name in"=w412, "error in"=w411, "Direction"=w414, "Server addr"=w413) -> ("Dispensed1"=w410:string, "VISA resource name out"=w409:refnum<visa-resource-name>, "error out"=w408:errorcluster)  [unwired: 5 in]
            "Dispensed4" <- w410
          }
        }
        n284 = Fract/Exp String To Number(string=w258) -> (number=w270:dbl)  [unwired: 3 in, 1 out]
        n285 = Subtract(x=w267, y=w270) -> (x-y=w269:dbl)
        n286 = Number To Fractional String(number=w269) -> (F-format string=w266:string)  [unwired: 3 in]
        n287 = Concatenate Strings(w266, "ML" ("string")) -> (→"Remains4":string)
        n288 = case shown="True" "Reset1" {
          tunnel: w256 -> [w397 w404]
          tunnel: w255 -> [w398 w403]
          tunnel: [w397 w400] -> w253
          tunnel: [w398 w399] -> w252
          frame False {
          }
          frame True {
            n289 = call "Function_reset.vi"("VISA resource name in"=w403, "error in"=w404, "Server addr"="0" ("trimmed string")) -> ("VISA resource name out"=w399:refnum<visa-resource-name>, "error out"=w400:errorcluster)  [unwired: 7 in]
            n290 = property on="Dispensed1" class="Str"("Value"="0" ("Vol Infused")) -> ()  [unwired: 2 in, 2 out]
          }
        }
        n291 = case shown="True" "Reset2" {
          tunnel: w253 -> [w389 w396]
          tunnel: w252 -> [w390 w395]
          tunnel: [w389 w392] -> w249
          tunnel: [w390 w391] -> w248
          frame False {
          }
          frame True {
            n292 = call "Function_reset.vi"("VISA resource name in"=w395, "error in"=w396, "Server addr"="1" ("trimmed string")) -> ("VISA resource name out"=w391:refnum<visa-resource-name>, "error out"=w392:errorcluster)  [unwired: 7 in]
            n293 = property on="Dispensed2" class="Str"("Value"="0" ("Vol Infused")) -> ()  [unwired: 2 in, 2 out]
          }
        }
        n294 = case shown="True" "Reset3" {
          tunnel: w249 -> [w382 w388]
          tunnel: w248 -> [w381 w383]
          tunnel: [w382 w385] -> w247
          tunnel: [w381 w384] -> w246
          frame False {
          }
          frame True {
            n295 = call "Function_reset.vi"("VISA resource name in"=w383, "error in"=w388, "Server addr"="2" ("trimmed string")) -> ("VISA resource name out"=w384:refnum<visa-resource-name>, "error out"=w385:errorcluster)  [unwired: 7 in]
            n296 = property on="Dispensed3" class="Str"("Value"="0" ("Vol Infused")) -> ()  [unwired: 2 in, 2 out]
          }
        }
        n297 = case shown="True" "Reset4" {
          tunnel: w247 -> [w373 w380]
          tunnel: w246 -> [w374 w379]
          tunnel: [w374 w376] -> w232
          tunnel: [w373 w375] -> w231
          frame False {
          }
          frame True {
            n298 = call "Function_reset.vi"("VISA resource name in"=w379, "error in"=w380, "Server addr"="3" ("trimmed string")) -> ("VISA resource name out"=w376:refnum<visa-resource-name>, "error out"=w375:errorcluster)  [unwired: 7 in]
            n299 = property on="Dispensed4" class="Str"("Value"="0" ("Vol Infused")) -> ()  [unwired: 2 in, 2 out]
          }
        }
      }
      n300 = xnode "Close FPGA VI Reference"("FPGA VI Reference In"=w64, "error in"=w63) -> ()  [unwired: 1 out]
      n301 = VISA Close(VISA resource name=w43, error in (no error)=w47) -> (error out=w48:errorcluster)
      n302 = call <vilib>:"Simple Error Handler.vi"("error in (no error)"=w48) -> ()  [unwired: 4 in, 5 out]
      n303 = VISA Close(VISA resource name=w52, error in (no error)=w51) -> (error out=w53:errorcluster)
      n304 = call <vilib>:"Simple Error Handler.vi"("error in (no error)"=w53) -> ()  [unwired: 4 in, 5 out]
      "Baud Rate" <- w56
    }
    frame #2 {
      n305 = local read "Data File Ptr"() -> (w774:refnum<file>)
      n306 = Close File(refnum=w774) -> ()  [unwired: 1 in, 2 out]
    }
  }
